vi "Multiple acquisition device control.vi"(1 "Number of acq. devs.":i32=3) -> (0 "Error Out":errorcluster)   [LabVIEW 2017]
uses:
  Sub VIs/Rendezvous global.vi
panel:
  out "End":bool
  out "Trigger set":bool
  out "Waiting for acq. devs.":bool
  # "Objective:\nGet all N acquisition devices configured ready for an external hardware trigger, and only set the trigger once they are ALL ready."
  # "PN 04/05/18"
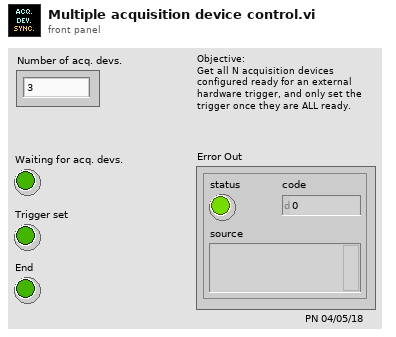
[diagram p1: front panel]
types:
  T1 = typedef "Rendezvous RefNum" = refnum<k1>
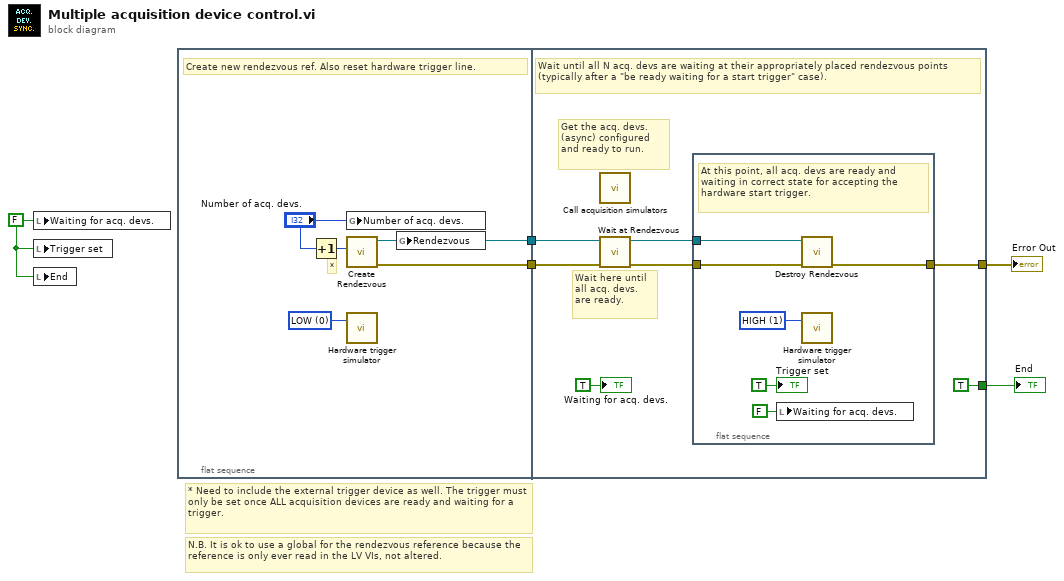
[diagram p0: block diagram]
diagram:
  w1 = FALSE ("Waiting for acq. devs.")
  # "N.B. It is ok to use a global for the rendezvous reference because the reference is only ever read in the LV VIs, not altered."
  # "* Need to include the external trigger device as well. The trigger must only be set once ALL acquisition devices are ready and waiting for a trigger."
  n1 = local write "Waiting for acq. devs."(w1) -> ()
  n2 = local write "Trigger set"(w1) -> ()
  n3 = local write "End"(w1) -> ()
  n4 = flat-sequence {
    tunnel: [w10] -> w5
    tunnel: [w8] -> w3
    tunnel: w5 -> [w16]
    tunnel: [w17] -> w4
    tunnel: w3 -> [w13]
    tunnel: [TRUE ("Setting trigger")] -> w2
    frame #0 {
      w9 = u8 0 items=["LOW", "HIGH"] ("State")
      # "*"
      # "Create new rendezvous ref. Also reset hardware trigger line."
      n5 = Increment(x="Number of acq. devs.") -> (x+1=w7:i32)
      n6 = global write "Rendezvous global.vi" "Number of acq. devs."("Number of acq. devs.") -> ()
      n7 = call <vilib>:"Create Rendezvous.vi"("size (2)"=w7) -> ("error out"=w10:errorcluster, "rendezvous"=w8:T1)  [unwired: 4 in, 1 out]
      n8 = call "Hardware trigger simulator.vi"("State"=w9) -> ()  [unwired: 3 in]
      n9 = global write "Rendezvous global.vi" "Rendezvous"(w8) -> ()
    }
    frame #1 {
      # "Wait here until all acq. devs. are ready."
      # "Get the acq. devs. (async) configured and ready to run."
      # "Wait until all N acq. devs are waiting at their appropriately placed rendezvous points (typically after a \"be ready waiting for a start trigger\" case)."
      n10 = call "Call acquisition simulators.vi"() -> ()  [unwired: 1 in]
      n11 = call <vilib>:"Wait at Rendezvous.vi"("error in (no error)"=w16, "rendezvous"=w13) -> ("error out"=w15:errorcluster, "rendezvous out"=w14:T1)  [unwired: 3 in, 1 out]
      n12 = flat-sequence {
        tunnel: w14 -> [w23]
        tunnel: w15 -> [w22]
        tunnel: [w20] -> w17
        frame #0 {
          w21 = u8 1 items=["LOW", "HIGH"] ("State")
          # "At this point, all acq. devs are ready and waiting in correct state for accepting the hardware start trigger."
          n13 = local write "Waiting for acq. devs."(FALSE ("Waiting for acq. devs.")) -> ()
          n14 = call <vilib>:"Destroy Rendezvous.vi"("error in (no error)"=w22, "rendezvous"=w23) -> ("error out"=w20:errorcluster)  [unwired: 4 in, 1 out]
          n15 = call "Hardware trigger simulator.vi"("State"=w21) -> ()  [unwired: 3 in]
          "Trigger set" <- TRUE ("Setting trigger")
        }
      }
      "Waiting for acq. devs." <- TRUE ("Waiting for acq. devs.")
    }
  }
  "Error Out" <- w4
  "End" <- w2
